vi "Write state.vi"(8 "error in (no error)":errorcluster, 10 "state":bool, 11 "Change Speaker State CMD in":refnum<class "Change Speaker State CMD.lvclass">) -> (0 "error out":errorcluster, 3 "Change Speaker State CMD out":refnum<class "Change Speaker State CMD.lvclass">)   [LabVIEW 2017, in "PAS Library.lvlib" / "Change Speaker State CMD.lvclass"]
uses:
  Change Speaker State CMD.lvclass
  Change Speaker State CMD.lvclass/Change Speaker State CMD.ctl
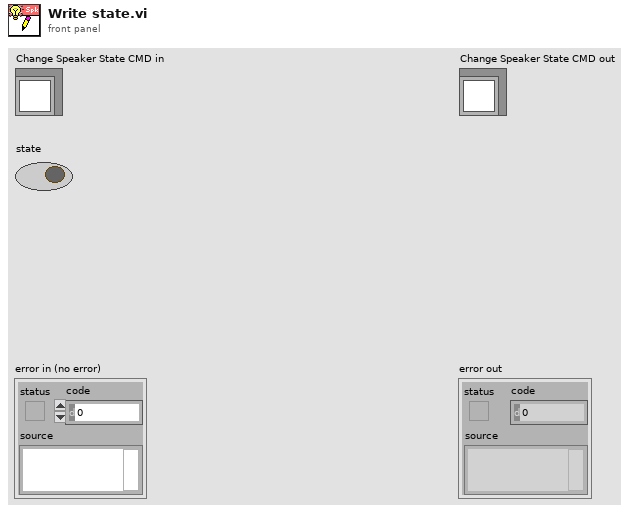
[diagram p1: front panel]
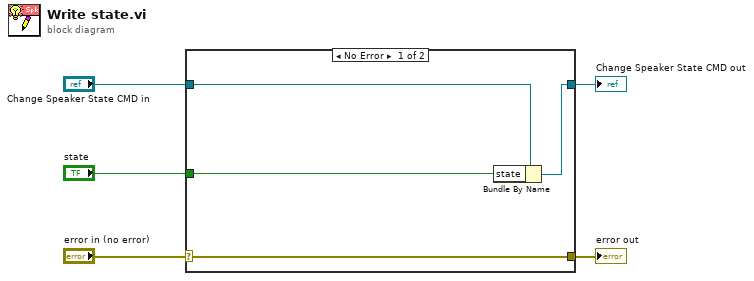
[diagram p0: block diagram]
diagram:
  n1 = case shown="No Error" "error in (no error)" {
    selector: "error in (no error)" -> [w9 w10]
    tunnel: [w9 w10] -> w4
    tunnel: [w7 w11] -> w2
    tunnel: "Change Speaker State CMD in" -> [w8 w11]
    tunnel: "state" -> [w6 _]
    frame No Error {
      n2 = Bundle By Name(cluster=w8, "state"=w6) -> (w7:refnum<class "Change Speaker State CMD.lvclass">)
    }
    frame Error {
    }
  }
  "error out" <- w4
  "Change Speaker State CMD out" <- w2
